vi "Rohde & Schwarz VNA Set Trace Status.vi"(4 "Trace":i32=1 min=1 max=99 step=1, 6 "Channel":i32=1 min=1 max=99 step=1, 7 "Rohde & Schwarz VNA":T1, 8 "error in (no error)":errorcluster, 11 "VISA Resource Name":refnum<visa-resource-name>) -> (0 "error out":errorcluster, 3 "dup VISA Resource Name":refnum<visa-resource-name>)   [LabVIEW 2011]
uses:
  TypeDefs/Rohde & Schwarz VNA Instrument Info.ctl
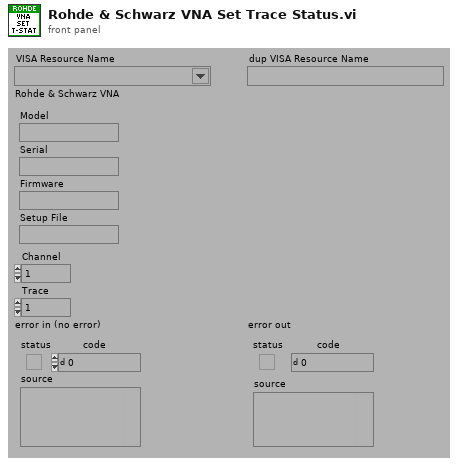
[diagram p1: front panel]
types:
  T1 = typedef "Rohde & Schwarz VNA Instrument Info.ctl" = cluster{"Model":string, "Serial":string, "Firmware":string, "Setup File":string}
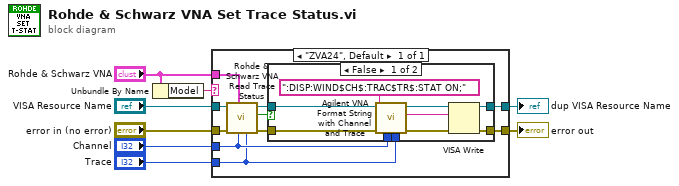
[diagram p0: block diagram]
diagram:
  n1 = Unbundle By Name("Rohde & Schwarz VNA") -> ("Model"=w1:string)
  n2 = case shown="\"ZVA24\", Default" w1 {
    tunnel: "VISA Resource Name" -> [w15]
    tunnel: "error in (no error)" -> [w16]
    tunnel: [w18] -> w6
    tunnel: [w17] -> w5
    tunnel: "Channel" -> [w11]
    tunnel: "Rohde & Schwarz VNA" -> [w12]
    tunnel: "Trace" -> [w10]
    frame "ZVA24", Default {
      n3 = call "Rohde & Schwarz VNA Read Trace Status.vi"("Trace"=w10, "Channel"=w11, "Rohde & Schwarz VNA"=w12, "error in (no error)"=w16, "VISA Resource Name"=w15) -> ("error out"=w13:errorcluster, "On?"=w9:bool, "dup VISA Resource Name"=w14:refnum<visa-resource-name>)  [unwired: 4 out]
      n4 = case shown="False" w9 {
        tunnel: [w26 w28] -> w18
        tunnel: [w25 w27] -> w17
        tunnel: w14 -> [w24 w28]
        tunnel: w13 -> [w23 w27]
        tunnel: w11 -> [w20 _]
        tunnel: w10 -> [w19 _]
        frame False {
          n5 = call "Agilent VNA Format String with Channel and Trace.vi"("Trace"=w19, "Channel"=w20, "String"=":DISP:WIND$CH$:TRAC$TR$:STAT ON;" ("write buffer")) -> ("String Out"=w22:string)  [unwired: 6 out]
          n6 = VISA Write(VISA resource name=w24, write buffer=w22, error in (no error)=w23) -> (VISA resource name out=w26:refnum<visa-resource-name>, error out=w25:errorcluster)  [unwired: 1 out]
        }
        frame True {
        }
      }
    }
  }
  "dup VISA Resource Name" <- w6
  "error out" <- w5
